vi "360 Angle Calc With Offset.vi"(11 "Center":cluster{"X":dbl, "Y":dbl}) -> (3 "angle":dbl)   [LabVIEW 2025]
panel:
  in  "deg/pix":dbl=0.125
  out "X":dbl
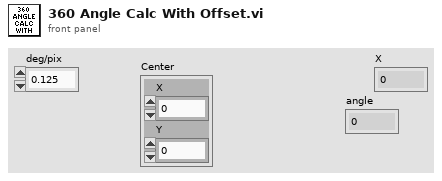
[diagram p1: front panel]
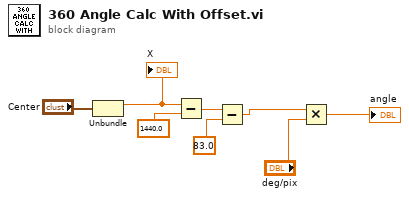
[diagram p0: block diagram]
diagram:
  n1 = Unbundle("Center") -> ("X"=w7:dbl)  [unwired: 1 out]
  "X" <- w7
  n2 = Subtract(x=w7, y=1440.0) -> (x-y=w3:dbl)
  n3 = Subtract(x=w3, y=83.0) -> (x-y=w1:dbl)
  n4 = Multiply(x=w1, y="deg/pix") -> (x*y=→"angle":dbl)
